vi "DAQ@WaveFormLoad__Parameter.vi"(1 "ParamterIn":string) -> (0 "ParamterOut":string)   [LabVIEW 2019]
uses:
  MainFrame/Global.vi
panel:
  in  "File":string(combo)
  in  "WaveFormName":string(combo)
  in  "Confirm":bool
  # "DAQ@WaveFormRead/WaveFormWrite $DAQ,$FileName"
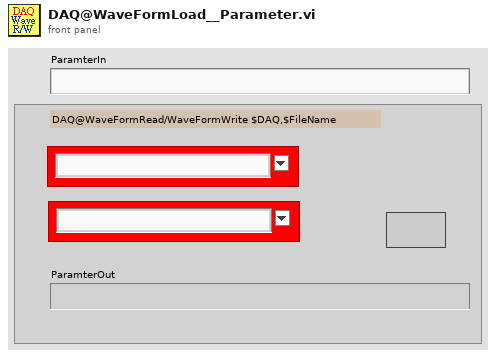
[diagram p1: front panel]
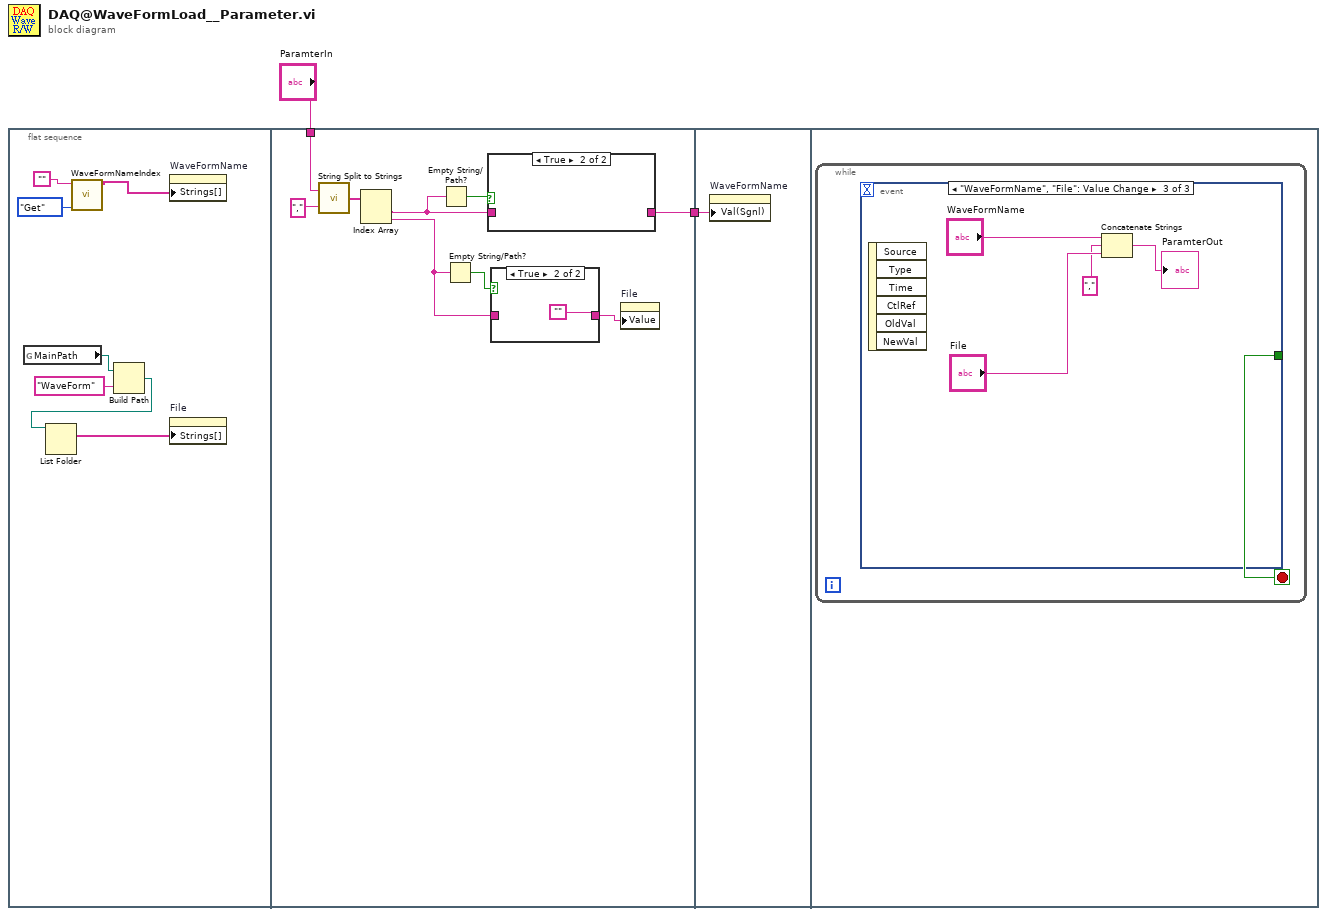
[diagram p0: block diagram]
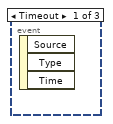
[diagram p4: hidden frame]
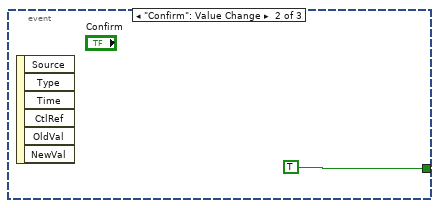
[diagram p5: hidden frame]
diagram:
  n1 = flat-sequence {
    tunnel: "ParamterIn" -> [w15]
    tunnel: [w10] -> w1
    tunnel: w1 -> [w22]
    frame #0 {
      n2 = global read "Global.vi" "MainPath"() -> (w6:path)
      n3 = call "WaveFormNameIndex.vi"("OP"=enum16{"Get", "Update", "Init", "GetSPS"}."Get", "WaveFormName"="") -> ("WaveFormNameList"=w7:string[])  [unwired: 6 in, 3 out]
      n4 = Build Path(base path=w6, name or relative path="WaveForm") -> (appended path=w4:path)
      n5 = List Folder(path=w4) -> (filenames=w3:string[])  [unwired: 3 in, 3 out]
      n6 = property on="WaveFormName" class="CmbBox"("Strings[]"=w7) -> ()  [unwired: 2 in, 2 out]
      n7 = property on="File" class="CmbBox"("Strings[]"=w3) -> ()  [unwired: 2 in, 2 out]
    }
    frame #1 {
      n8 = call "String Split to Strings.vi"("search string/char (-)"=",", "String"=w15) -> ("Array"=w17:string[])
      n9 = Index Array(array=w17) -> (element #1=w14:string, element #2=w11:string)  [unwired: 2 in]
      n10 = Empty String/Path?(string/path=w14) -> (empty?=w18:bool)
      n11 = Empty String/Path?(string/path=w11) -> (empty?=w13:bool)
      n12 = case shown="True" w18 {
        tunnel: w14 -> [w21 _]
        tunnel: [w21 _] -> w10
        frame False {
        }
        frame True {
        }
      }
      n13 = case shown="True" w13 {
        tunnel: [w19 ""] -> w12
        tunnel: w11 -> [w19 _]
        frame False {
        }
        frame True {
        }
      }
      n14 = property on="File" class="CmbBox"("Value"=w12) -> ()  [unwired: 2 in, 2 out]
    }
    frame #2 {
      n15 = property on="WaveFormName" class="CmbBox"("Val(Sgnl)"=w22) -> ()  [unwired: 2 in, 2 out]
    }
    frame #3 {
      n16 = while {
        stop <- w23 stop-if-true
        n17 = event shown="[2] \"WaveFormName\", \"File\": Value Change" {
          selector: _ -> [_ _ _]
          dyn-events: _ -> [_ _ _]
          timeout: _ -> [_ _ _]
          tunnel: [_ TRUE _] -> w23
          event Timeout {
            n18 = event-data() -> ()  [unwired: 1 in, 3 out]
          }
          event "Confirm": Value Change {
            n19 = event-data() -> ()  [unwired: 1 in, 6 out]
          }
          event "WaveFormName", "File": Value Change {
            n20 = event-data() -> ()  [unwired: 1 in, 6 out]
            n21 = Concatenate Strings("WaveFormName", ",", "File") -> (→"ParamterOut":string)
          }
        }
      }
    }
  }
